vi "Untitled 1 (SubVI).vi"(5 "Imp Type (0: CPD)":u32(ring)=15 items=["CPD", "CPQ", "CPG", "CPRP", "CSD", "CSQ", "CSRS", "LPQ", "LPD", "LPG", "LPRP", "LSD", "LSQ", "LSRS", "RX", "ZTD", "ZTR", "GB", "YTD", "YTR"], 6 "Bias(mA)":dbl=60.0 format="%#_13g", 7 "Current Level (mA)":dbl=10.0 format="%#_13g", 8 "error in (no error)":errorcluster, 9 "Frecuency (KHz)":dbl=250.0 format="%#_13g", 10 "Voltage (V)(1.0V)":dbl=1.0 min=0.0 max=20.0 step=0.1 format="%.4f", 11 "VISA Refnum in":refnum<visa-resource-name>="GPIB0::17::INSTR") -> (0 "error out":errorcluster, 3 "VISA Refnum out":refnum<visa-resource-name>)   [LabVIEW 2015]
uses:
  <instrlib>/Agilent 428X Series/Agilent 428X Series.lvlib
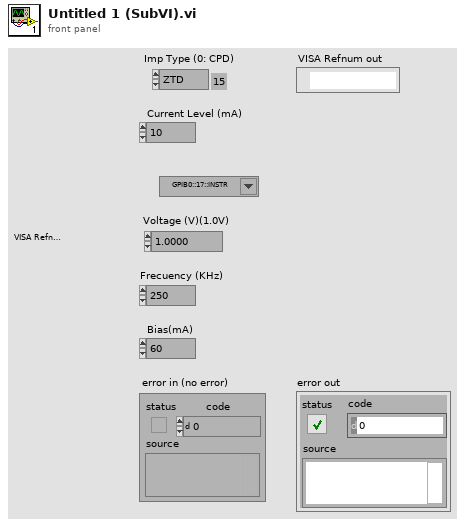
[diagram p1: front panel]
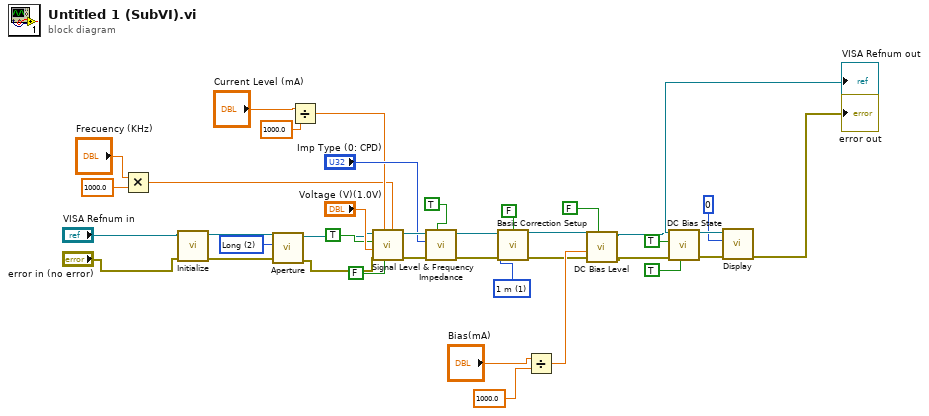
[diagram p0: block diagram]
diagram:
  w6 = u32 1 items=["0 m", "1 m", "2 m", "3 m", "4 m"] ("Cable Length (0: 4 m)")
  w12 = u32 2 items=["Short", "Medium", "Long"] ("Integ Time (0: Short)")
  n1 = Multiply(x="Frecuency (KHz)", y=1000.0) -> (x*y=w21:dbl)
  n2 = call <instrlib>:"Initialize.vi"("error in (no error)"="error in (no error)", "VISA resource name"="VISA Refnum in") -> ("error out"=w13:errorcluster, "VISA resource name out"=w14:refnum<visa-resource-name>)  [unwired: 8 in]
  n3 = call <instrlib>:"Aperture.vi"("error in (no error)"=w13, "Integ Time (0: Short)"=w12, "VISA resource name"=w14) -> ("error out"=w10:errorcluster, "VISA resource name out"=w11:refnum<visa-resource-name>)  [unwired: 7 in]
  n4 = Divide(x="Current Level (mA)", y=1000.0) -> (x/y=w26:dbl)
  n5 = call <instrlib>:"Signal Level & Frequency.vi"("Frequency Value (Hz) (100KHz)"=w21, "Oscillator Select (T: Voltage)"=FALSE, "Current Level (A) (100uA)"=w26, "error in (no error)"=w10, "Voltage Level (V) (5mV)"="Voltage (V)(1.0V)", "Auto Level Control (F: Off)"=TRUE, "VISA resource name"=w11) -> ("error out"=w36:errorcluster, "VISA resource name out"=w37:refnum<visa-resource-name>)  [unwired: 3 in]
  n6 = call <instrlib>:"Impedance.vi"("Auto Range (F: Off)"=TRUE ("Auto Range (Off:F)"), "error in (no error)"=w36, "Imp Type (0: CPD)"="Imp Type (0: CPD)", "VISA resource name"=w37) -> ("error out"=w2:errorcluster, "VISA resource name out"=w4:refnum<visa-resource-name>)  [unwired: 6 in]
  n7 = call <instrlib>:"Basic Correction Setup.vi"("VISA resource name"=w4, "Short Corr (T: On)"=FALSE, "Cable Length (0: 4 m)"=w6, "error in (no error)"=w2) -> ("VISA resource name out"=w3:refnum<visa-resource-name>, "error out"=w1:errorcluster)  [unwired: 9 in, 1 out]
  n8 = Divide(x="Bias(mA)", y=1000.0) -> (x/y=w23:dbl)
  n9 = call <instrlib>:"DC Bias Level.vi"("Level Selector (T: Volt)"=FALSE, "error in (no error)"=w1, "Current Level (A) (0.0)"=w23, "VISA resource name"=w3) -> ("error out"=w7:errorcluster, "VISA resource name out"=w8:refnum<visa-resource-name>)  [unwired: 6 in]
  n10 = call <instrlib>:"DC Bias State.vi"("Curr Bias Monitor (F: Off)"=TRUE, "error in (no error)"=w7, "State (F: Off)"=TRUE, "VISA resource name"=w8) -> ("error out"=w20:errorcluster, "VISA resource name out"=w19:refnum<visa-resource-name>)  [unwired: 6 in]
  n11 = call <instrlib>:"Display.vi"("error in (no error)"=w20, "Display Page (0: Measurement)"=u32 0 ("Display Page (Measurment:0)"), "VISA resource name"=w19) -> ("error out"=→"error out":errorcluster, "VISA resource name out"=→"VISA Refnum out":refnum<visa-resource-name>)  [unwired: 7 in]
